vi "configure.vi"(8 "error in (no error)":errorcluster, 11 "YK090623DAQmxAnalogDetector in":refnum<class "DetectorYK090623DAQmxAnalog.lvclass">) -> (0 "error out":errorcluster, 3 "YK090623DAQmxAnalogDetector out":refnum<class "DetectorYK090623DAQmxAnalog.lvclass">)   [LabVIEW 2010, in "DetectorYK090623DAQmxAnalog.lvclass"]
doc: "The dynamic dispatch version of this VI loads and displays the configuration file associated with the plug-in object. The user modify and save the configuration data."
uses:
  DetectorYK090623DAQmxAnalog.lvclass
  common/xcontrols/XComponentSpecification/XComponentSpecification/XComponentSpecification.xctl
  DetectorYK090623DAQmxAnalog.lvclass/DetectorYK090623DAQmxAnalog.ctl
  common/classes/ErrorController/ErrorController/class_data.vi
  common/classes/GenericComponent/GenericComponent/GenericComponent.lvclass
  common/classes/ErrorController/ErrorController/ErrorController.lvclass
panel:
  in  "analogOut spec":T1(xcontrol)
  out "Configuration":string
  in  "Default voltage":dbl[unit]
  in  "cancel button":bool
  in  "save button":bool
  # "Configure DetectorYK090623Analog"
  # "AnalogOut component"
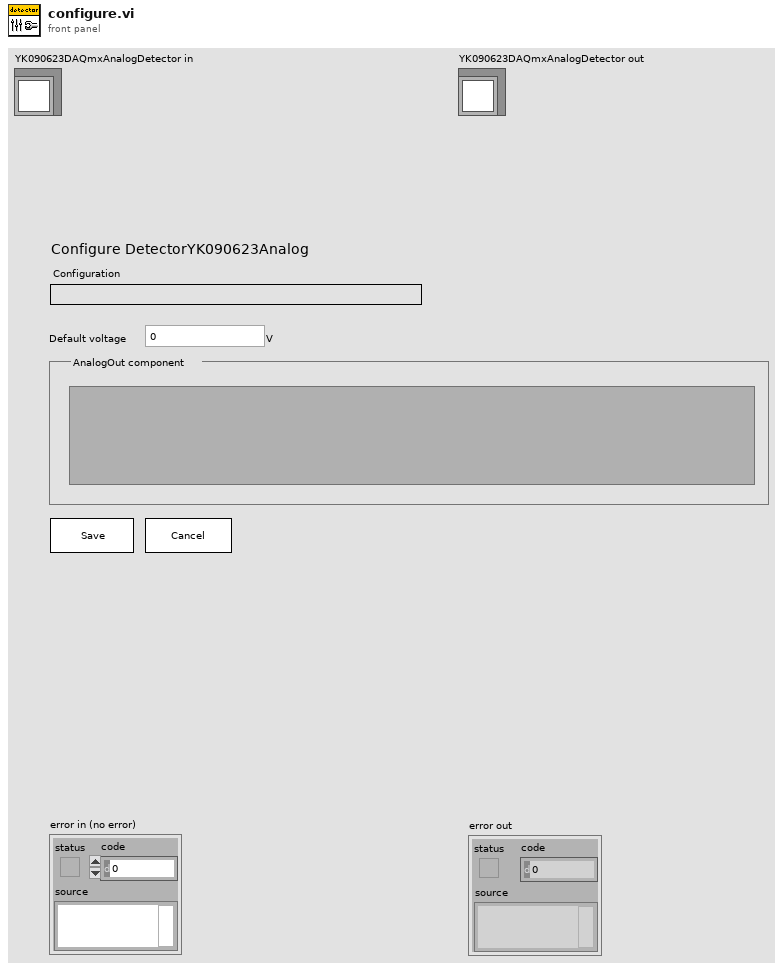
[diagram p1: front panel]
types:
  T1 = cluster{"class path":string, "configuration":string, "label":string, "settings name":string}
  T2 = typedef "plugin_specification.ctl" = cluster{"class path":string, "configuration":string, "label":string, "settings name":string}
  T3 = typedef "DetectorYK090623DAQmxAnalog.lvclass/config_data_cluster.ctl" = cluster{"default voltage":dbl[unit], "analog out":T2}
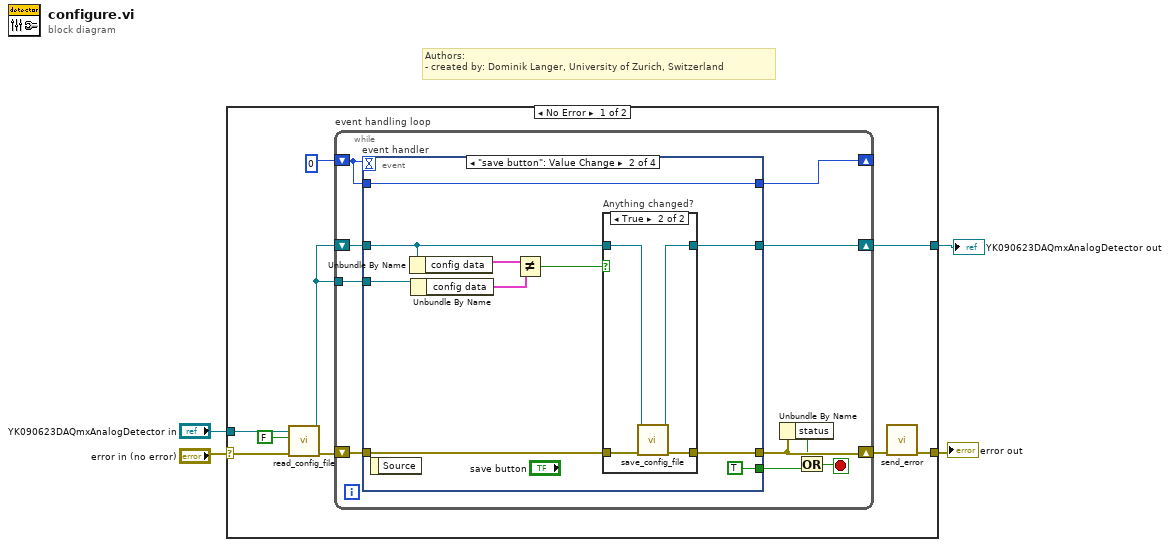
[diagram p0: block diagram]
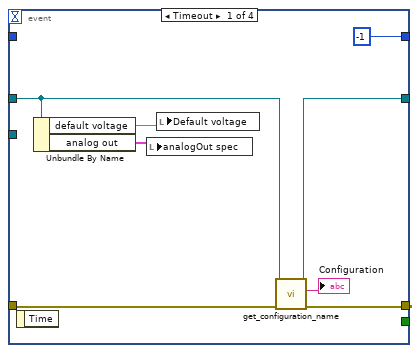
[diagram p2: hidden frame]
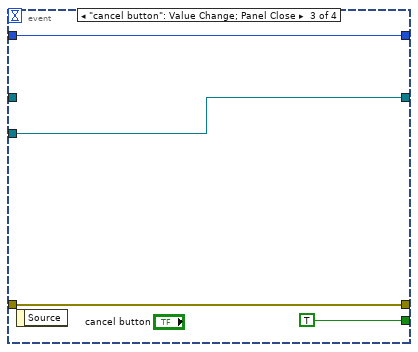
[diagram p4: hidden frame]
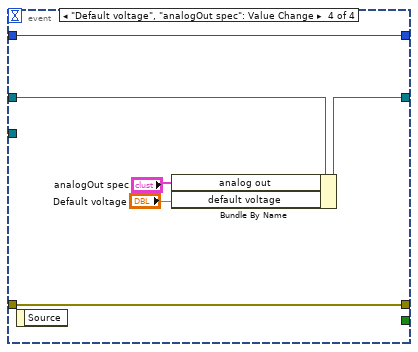
[diagram p5: hidden frame]
diagram:
  # "Authors: \n- created by: Dominik Langer, University of Zurich, Switzerland"
  n1 = case shown="No Error" "error in (no error)" {
    selector: "error in (no error)" -> [w13 w59]
    tunnel: [w6 w59] -> w3
    tunnel: "YK090623DAQmxAnalogDetector in" -> [w11 w58]
    tunnel: [w9 w58] -> w1
    frame No Error {
      n2 = call-dynamic "read_config_file.vi"("error in (no error)"=w13, "force load?"=FALSE, "GenericPlugin in"=w11) -> ("error out"=w12:errorcluster, "GenericPlugin out"=w7:refnum<class "DetectorYK090623DAQmxAnalog.lvclass">)  [unwired: 7 out]
      n3 = while "event handling loop" {
        shift-right: [w21] -> w9
        shift-left: w7 -> [w22]
        shift-right: [w14] -> _
        shift-left: 0 -> [w20]
        tunnel: w7 -> [w19]
        shift-right: [w18] -> w5
        shift-left: w12 -> [w23]
        stop <- w15 stop-if-true
        n4 = event "event handler" shown="[1] \"save button\": Value Change" {
          selector: _ -> [_ _ _ _]
          dyn-events: _ -> [_ _ _ _]
          timeout: w20 -> [_ _ _ _]
          tunnel: w23 -> [w25 w39 w51 w55]
          tunnel: [w29 w33 w51 w55] -> w18
          tunnel: w22 -> [w24 w37 _ w53]
          tunnel: [w27 w32 w48 w52] -> w21
          tunnel: [_ TRUE TRUE _] -> w17
          tunnel: [-1 w40 w49 w57] -> w14
          tunnel: w20 -> [_ w40 w49 w57]
          tunnel: w19 -> [_ w35 w48 _]
          event Timeout {
            n5 = event-data() -> ()  [unwired: 2 out]
            n6 = Unbundle By Name(w24) -> ("default voltage"=w30:dbl[unit], "analog out"=w26:T2)
            n7 = local write "analogOut spec"(w26) -> ()
            n8 = local write "Default voltage"(w30) -> ()
            n9 = call "get_configuration_name.vi"("error in (no error)"=w25, "GenericPlugin.lvclass in"=w24) -> ("error out"=w29:errorcluster, "configuration name"=→"Configuration":string, "GenericPlugin.lvclass out"=w27:refnum<class "DetectorYK090623DAQmxAnalog.lvclass">)  [unwired: 7 in]
          }
          event "save button": Value Change {
            n10 = event-data() -> ()  [unwired: 2 out]
            n11 = Unbundle By Name(w37) -> ("config data"=w36:T3)
            n12 = Unbundle By Name(w35) -> ("config data"=w34:T3)
            n13 = Not Equal?(x=w36, y=w34) -> (x != y?=w38:bool)
            n14 = case "Anything changed?" shown="True" w38 {
              tunnel: w39 -> [w43 w47]
              tunnel: [w43 w46] -> w33
              tunnel: w37 -> [w42 w44]
              tunnel: [w42 w45] -> w32
              frame False {
              }
              frame True {
                n15 = call-dynamic "save_config_file.vi"("error in (no error)"=w47, "GenericPlugin in"=w44) -> ("error out"=w46:errorcluster, "GenericPlugin out"=w45:refnum<class "DetectorYK090623DAQmxAnalog.lvclass">)  [unwired: 1 in, 7 out]
              }
            }
          }
          event "cancel button": Value Change; Panel Close {
            n16 = event-data() -> ()  [unwired: 2 out]
          }
          event "Default voltage", "analogOut spec": Value Change {
            n17 = event-data() -> ()  [unwired: 2 out]
            n18 = Bundle By Name(cluster=w53, "analog out"="analogOut spec", "default voltage"="Default voltage") -> (w52:refnum<class "DetectorYK090623DAQmxAnalog.lvclass">)
          }
        }
        n19 = Unbundle By Name(w18) -> ("status"=w16:bool)
        n20 = Or(x=w16, y=w17) -> (x .or. y?=w15:bool)
      }
      n21 = call "send_error.vi"("error in (no error)"=w5) -> ("error out"=w6:errorcluster)  [unwired: 10 in]
    }
    frame Error {
    }
  }
  "error out" <- w3
  "YK090623DAQmxAnalogDetector out" <- w1
